vi "Translator Some Digital Filters Functions.vi"(0 "Input":variant=variant("Function Name"=variant(string "Strip Path"), "Input Datatypes"=variant(string[] ["error", "int"]), "Inputs"=variant(string[] ["error in", "x"]), "Node refnum"=variant(refnum<vi> refnum), "Output Datatypes"=variant(string[] ["int"]), "Outputs"=variant(string[] ["a"])), 11 "error in (no error)":errorcluster) -> (4 "Output":variant=variant("Defines"=variant(string[] []), "Includes"=variant(string[] []), "Replaced Code"=variant(string "/* LabVIEW system function 'Strip Path' not found. */")), 15 "error out":errorcluster)   [LabVIEW 2014, in "Digital Filter Library.lvlib"]
doc: "source: https://www.arduino.cc/en/Reference/SPIEnd\n\nDisables the SPI bus (leaving pin modes unchanged).\n\nSyntax\n SPI.end()\n\nParameters\n None\n\nReturns\n None"
uses:
  Digital Filter Library.lvlib
panel:
  out "Outputs":string[](array[string])
  out "Inputs":string[](array[string])
  out "Output Datatypes":string[](array[string])
  out "Input Datatypes":string[](array[string])
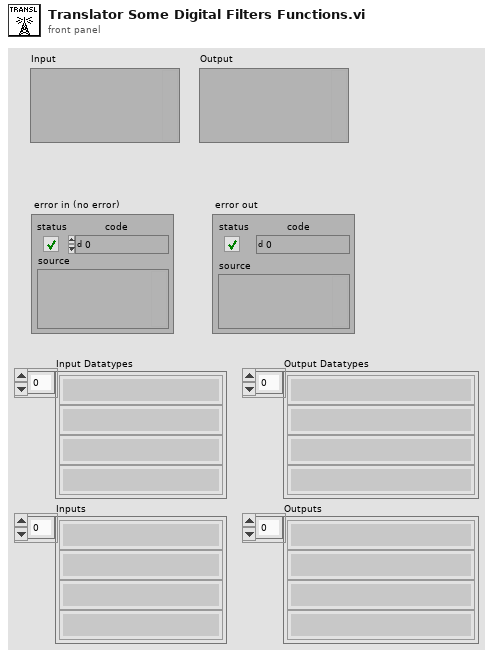
[diagram p1: front panel]
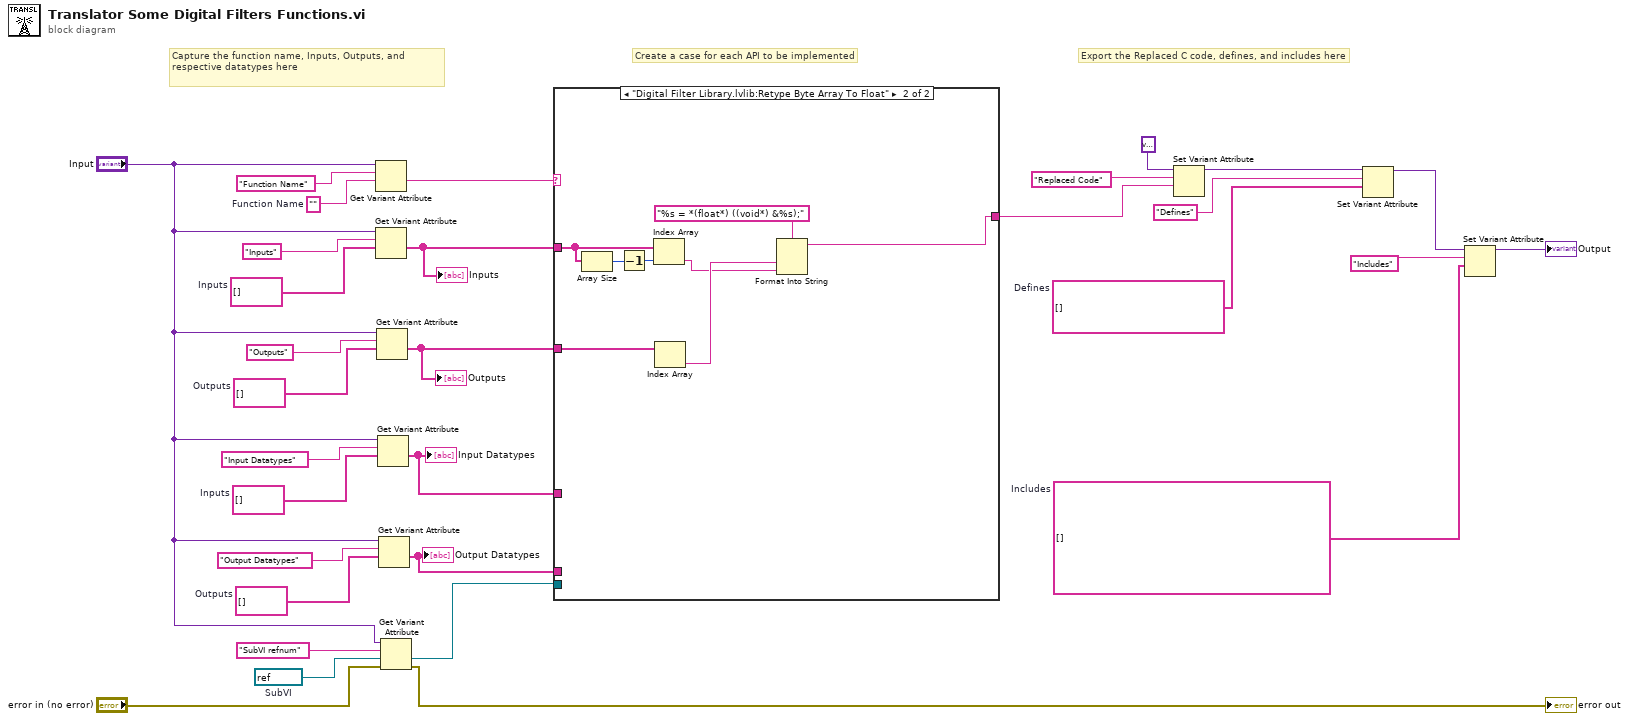
[diagram p0: block diagram]
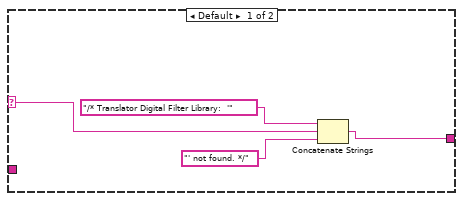
[diagram p2: hidden frame]
diagram:
  w7 = refnum<vi> refnum  # SubVI
  w4 = string[] []  # Defines
  w17 = string[] []  # Outputs
  w18 = string[] []  # Inputs
  w3 = string[] []  # Includes
  w27 = string[] []  # Outputs
  w28 = string[] []  # Inputs
  w29 = ""  # Function Name
  # "Capture the function name, Inputs, Outputs, and respective datatypes here"
  # "Export the Replaced C code, defines, and includes here"
  # "Create a case for each API to be implemented"
  n1 = Get Variant Attribute(Variant="Input", name="Function Name", default value (empty Variant)=w29) -> (value=w24:string)  [unwired: 1 in, 3 out]
  n2 = Get Variant Attribute(Variant="Input", name="Inputs", default value (empty Variant)=w28) -> (value=w14:string[])  [unwired: 1 in, 3 out]
  "Inputs" <- w14
  n3 = Get Variant Attribute(Variant="Input", name="Outputs", default value (empty Variant)=w27) -> (value=w15:string[])  [unwired: 1 in, 3 out]
  "Outputs" <- w15
  n4 = Get Variant Attribute(Variant="Input", name="Input Datatypes", default value (empty Variant)=w18) -> (value=w10:string[])  [unwired: 1 in, 3 out]
  "Input Datatypes" <- w10
  n5 = Get Variant Attribute(Variant="Input", name="Output Datatypes", default value (empty Variant)=w17) -> (value=w5:string[])  [unwired: 1 in, 3 out]
  "Output Datatypes" <- w5
  n6 = Get Variant Attribute(Variant="Input", name="SubVI refnum", default value (empty Variant)=w7, error in="error in (no error)") -> (value=w6:refnum<vi>, error out=→"error out":errorcluster)  [unwired: 2 out]
  n7 = case shown="\"Digital Filter Library.lvlib:Retype Byte Array To Float\"" w24 {
    selector: w24 -> [w34 _]
    tunnel: [w32 w38] -> w23
    tunnel: w14 -> [_ w36]
    tunnel: w15 -> [_ w43]
    tunnel: w10 -> [_ _]
    tunnel: w6 -> [_ _]
    tunnel: w5 -> [_ _]
    frame Default {
      n8 = Concatenate Strings("/* Translator Digital Filter Library:  '", w34, "' not found. */") -> (w32:string)
    }
    frame "Digital Filter Library.lvlib:Retype Byte Array To Float" {
      n9 = Array Size(array=w36) -> (size(s)=w42:i32)
      n10 = Decrement(x=w42) -> (x-1=w37:i32)
      n11 = Index Array(array=w36, index=w37) -> (element=w39:string)
      n12 = Index Array(array=w43) -> (element=w40:string)  [unwired: 1 in]
      n13 = Format Into String(format string="%s = *(float*) ((void*) &%s);", w40, w39) -> (resulting string=w38:string)  [unwired: 2 in, 1 out]
    }
  }
  n14 = Set Variant Attribute(Variant=variant ("variant"), name="Replaced Code", value=w23) -> (Variant out=w13:variant)  [unwired: 1 in, 2 out]
  n15 = Set Variant Attribute(Variant=w13, name="Defines", value=w4) -> (Variant out=w12:variant)  [unwired: 1 in, 2 out]
  n16 = Set Variant Attribute(Variant=w12, name="Includes", value=w3) -> (Variant out=→"Output":variant)  [unwired: 1 in, 2 out]
